vi "Authentication_Header_Handler.vi"(10 "String":string) -> (2 "output array":T1[](array[typedef]))   [LabVIEW 2016]
uses:
  <vilib>/addons/_JKI.lib/REST Client/classes/REST Client/HTTP Header.ctl
  <vilib>/addons/_JKI.lib/REST Client/classes/REST Client/REST Client.lvclass
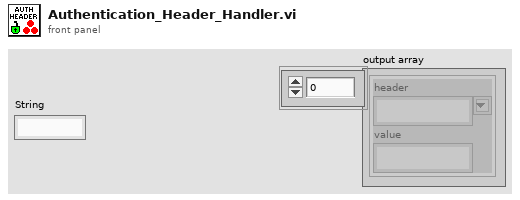
[diagram p1: front panel]
types:
  T1 = typedef "REST Client.lvlib/REST Client.lvclass/HTTP Header.ctl" = cluster{"header":string, "value":string}
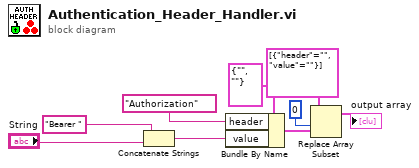
[diagram p0: block diagram]
diagram:
  n1 = Concatenate Strings("Bearer ", "String") -> (w6:string)
  n2 = Bundle By Name(cluster=T1 {"header"="", "value"=""} ("Header"), "header"="Authorization", "value"=w6) -> (w5:T1)
  n3 = Replace Array Subset(array=T1[] [{"header"="", "value"=""}] ("request specific headers"), new element=w5, index=0) -> (→"output array":T1[])
